vi "ConvertGoop3ToGoop4_RewireGetAttributes.vi"(8 "error in (no error)":errorcluster, 11 "ViRef":refnum<vi>) -> (0 "error out":errorcluster, 3 "ViRefOut":refnum<vi>)   [LabVIEW 2014]
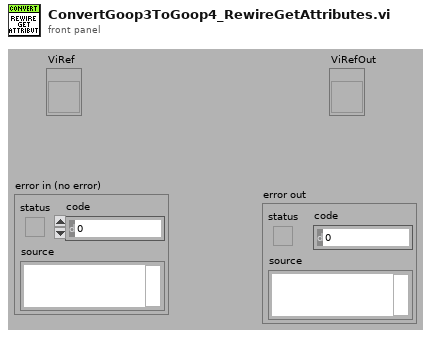
[diagram p1: front panel]
types:
  T1 = enum32{"invalid lock state", "Not Locked", "Locked (No Password)", "Password-protected"}
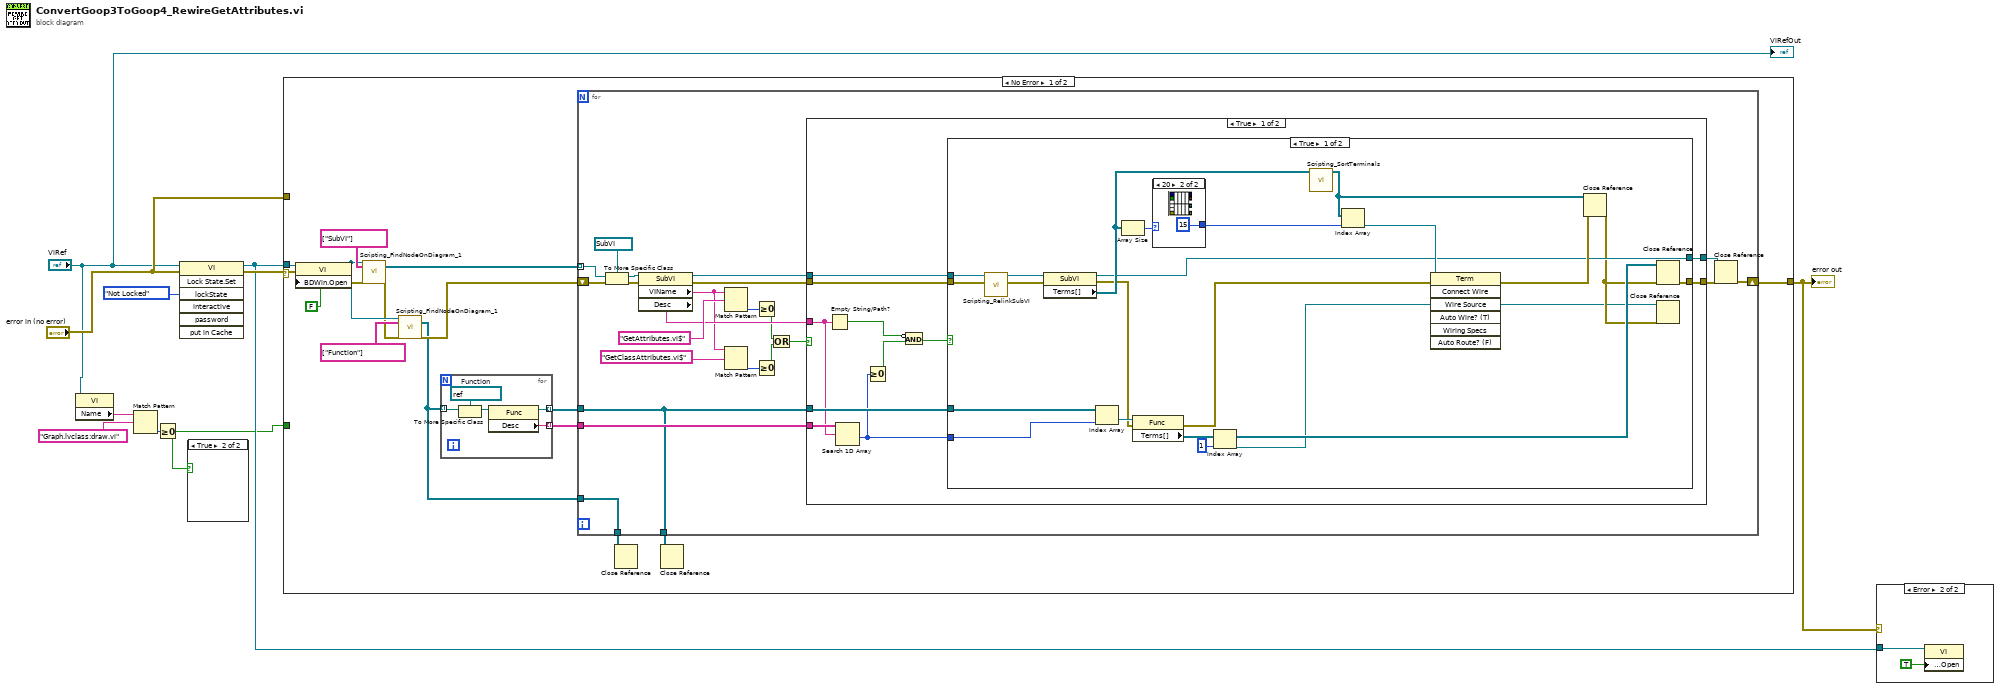
[diagram p0: block diagram]
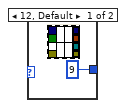
[diagram p4: hidden frame]
diagram:
  n1 = property class="VI"(reference="ViRef") -> ("Name"=w5:string)  [unwired: 1 in, 2 out]
  n2 = Match Pattern(string=w5, regular expression="Graph.lvclass:draw.vi") -> (offset past match=w3:i32)  [unwired: 1 in, 3 out]
  n3 = Greater Or Equal To 0?(x=w3) -> (x >= 0?=w1:bool)
  n4 = invoke class="VI" method="Lock State.Set"(reference="ViRef", error in="error in (no error)", "lockState"=T1."Not Locked" ("Lock State")) -> (reference out=w6:refnum<vi>, error out=w8:errorcluster)  [unwired: 4 in, 5 out]
  n5 = case shown="True" w1 {
    frame False {
    }
    frame True {
    }
  }
  n6 = case shown="No Error" w8 {
    selector: w8 -> [w21 _]
    tunnel: [w24 w92] -> w7
    tunnel: w6 -> [w22 _]
    tunnel: "error in (no error)" -> [_ w92]
    tunnel: w1 -> [_ _]
    frame No Error {
      n7 = property class="VI"(reference=w22, error in=w21, "BDWin.Open"=FALSE ("Block Diagram Window:Open")) -> (reference out=w20:refnum<vi>, error out=w23:errorcluster)
      n8 = call <resource>:"Scripting_FindNodeOnDiagram_1.vi"("ViRef(Ignored If Not Wired)"=w20, "NodeTypesToSearchFor"=string[] ["SubVI"], "error in (no error)"=w23) -> ("Nodes"=w25:refnum<vi>[], "error out"=w18:errorcluster)  [unwired: 15 in]
      n9 = call <resource>:"Scripting_FindNodeOnDiagram_1.vi"("ViRef(Ignored If Not Wired)"=w20, "NodeTypesToSearchFor"=string[] ["Function"], "error in (no error)"=w18) -> ("Nodes"=w13:refnum<vi>[], "error out"=w17:errorcluster)  [unwired: 15 in]
      n10 = for {
        tunnel: w13 -> [w29] mode=indexing
        tunnel: [w28] -> w16 mode=indexing
        tunnel: [w27] -> w15 mode=indexing
        w30 = refnum<vi> refnum  # Function
        n11 = To More Specific Class(target class=w30, reference=w29) -> (specific class reference=w31:refnum<vi>)  [unwired: 1 in, 1 out]
        n12 = property class="Func"(reference=w31) -> (reference out=w27:refnum<vi>, "Desc"=w28:string)  [unwired: 1 in, 1 out]
      }
      n13 = for {
        tunnel: w25 -> [w53] mode=indexing
        shift-right: [w44] -> w24
        shift-left: w17 -> [w51]
        tunnel: w16 -> [w42]
        tunnel: w15 -> [w41]
        tunnel: [w41] -> w14
        tunnel: w13 -> [w40]
        tunnel: [w40] -> w12
        n14 = To More Specific Class(target class=refnum<vi> refnum ("WhileLoop"), reference=w53, error in=w51) -> (specific class reference=w50:refnum<vi>, error out=w49:errorcluster)
        n15 = property class="SubVI"(reference=w50, error in=w49) -> (reference out=w47:refnum<vi>, error out=w46:errorcluster, "VIName"=w38:string, "Desc"=w39:string)
        n16 = Match Pattern(string=w38, regular expression="GetAttributes.vi$") -> (offset past match=w36:i32)  [unwired: 1 in, 3 out]
        n17 = Match Pattern(string=w38, regular expression="GetClassAttributes.vi$") -> (offset past match=w35:i32)  [unwired: 1 in, 3 out]
        n18 = Greater Or Equal To 0?(x=w36) -> (x >= 0?=w34:bool)
        n19 = Greater Or Equal To 0?(x=w35) -> (x >= 0?=w33:bool)
        n20 = Or(x=w34, y=w33) -> (x .or. y?=w32:bool)
        n21 = case shown="True" w32 {
          tunnel: w47 -> [w64 w90]
          tunnel: w46 -> [w63 w91]
          tunnel: [w62 w91] -> w45
          tunnel: w39 -> [w58 _]
          tunnel: [w59 w90] -> w43
          tunnel: w42 -> [w61 _]
          tunnel: w41 -> [w60 _]
          frame True {
            n22 = Empty String/Path?(string/path=w58) -> (empty?=w57:bool)
            n23 = Search 1D Array(1D array=w61, element=w58) -> (index of element=w55:i32)  [unwired: 1 in]
            n24 = Greater Or Equal To 0?(x=w55) -> (x >= 0?=w56:bool)
            n25 = Compound Arithmetic op=AND(invert w57, w56) -> (w54:bool)
            n26 = case shown="True" w54 {
              tunnel: w64 -> [w69 w89]
              tunnel: w63 -> [w68 w88]
              tunnel: [w80 w88] -> w62
              tunnel: w60 -> [w79 _]
              tunnel: [w77 w89] -> w59
              tunnel: w55 -> [w65 _]
              frame True {
                n27 = call <resource>:"Scripting_RelinkSubVI.vi"("error in"=w68, "SubVIIn"=w69) -> ("error out"=w66:errorcluster, "SubVIOut"=w67:refnum<vi>)  [unwired: 8 in]
                n28 = property class="SubVI"(reference=w67, error in=w66) -> (reference out=w77:refnum<vi>, error out=w75:errorcluster, "Terms[]"=w85:refnum<vi>[])
                n29 = Index Array(array=w79, index=w65) -> (element=w76:refnum<vi>)
                n30 = Array Size(array=w85) -> (size(s)=w84:i32)
                n31 = property class="Func"(reference=w76, error in=w75) -> (error out=w73:errorcluster, "Terms[]"=w72:refnum<vi>[])  [unwired: 1 out]
                n32 = case shown="20" w84 {
                  tunnel: [9 ("index") 15 ("index")] -> w83
                  frame 12, Default {
                  }
                  frame 20 {
                  }
                }
                n33 = Index Array(array=w72, index=1) -> (element=w70:refnum<vi>)
                n34 = call <resource>:"Scripting_SortTerminals.vi"("Terminals[]"=w85) -> ("TerminalsOut[]"=w82:refnum<vi>[])  [unwired: 8 in, 2 out]
                n35 = Index Array(array=w82, index=w83) -> (element=w78:refnum<vi>)
                n36 = invoke class="Term" method="Connect Wire"(reference=w78, error in=w73, "Wire Source"=w70) -> (error out=w81:errorcluster)  [unwired: 4 in, 6 out]
                n37 = Close Reference(reference=w82, error in (no error)=w81) -> (error out=w71:errorcluster)
                n38 = Close Reference(reference=w72, error in (no error)=w71) -> (error out=w80:errorcluster)
                n39 = Close Reference(reference=w70, error in (no error)=w71) -> ()  [unwired: 1 out]
              }
              frame False {
              }
            }
          }
          frame False {
          }
        }
        n40 = Close Reference(reference=w43, error in (no error)=w45) -> (error out=w44:errorcluster)
      }
      n41 = Close Reference(reference=w12) -> ()  [unwired: 1 in, 1 out]
      n42 = Close Reference(reference=w14) -> ()  [unwired: 1 in, 1 out]
    }
    frame Error {
    }
  }
  "error out" <- w7
  n43 = case shown="Error" w7 {
    tunnel: w6 -> [_ w93]
    frame No Error {
    }
    frame Error {
      n44 = property class="VI"(reference=w93, "Front Panel.Open"=TRUE ("Front Panel Window:Open")) -> ()  [unwired: 1 in, 2 out]
    }
  }
  "ViRefOut" <- "ViRef"
